vi "ShoulderGetSetpointPreset.vi"(8 "SholdrSetpoints":T1=enum."ShoulderAmp") -> (0 "Setpoint":dbl)   [LabVIEW 2023]
doc: "Gets arm position depending enum value"
uses:
  ShoulderGetSetpointEnum.ctl
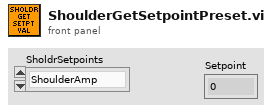
[diagram p1: front panel]
types:
  T1 = typedef "ShoulderGetSetpointEnum.ctl" = enum16{"ShoulderRest", "ShoulderSpeaker", "ShoulderAmp"}
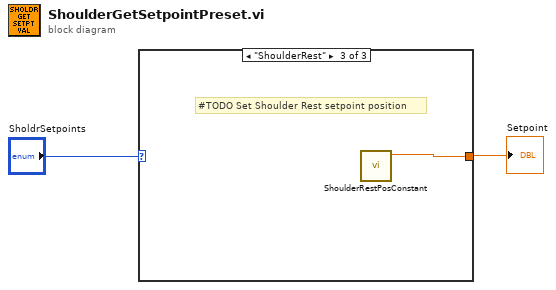
[diagram p0: block diagram]
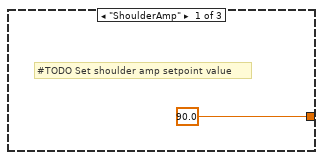
[diagram p2: hidden frame]
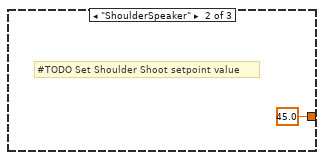
[diagram p3: hidden frame]
diagram:
  n1 = case shown="\"ShoulderRest\"" "SholdrSetpoints" {
    tunnel: [90.0 ("y") 45.0 ("y") w5] -> w1
    frame "ShoulderAmp" {
      # "#TODO Set shoulder amp setpoint value"
    }
    frame "ShoulderSpeaker" {
      # "#TODO Set Shoulder Shoot setpoint value"
    }
    frame "ShoulderRest" {
      # "#TODO Set Shoulder Rest setpoint position"
      n2 = call "ShoulderRestPosConstant.vi"() -> ("RestPosition"=w5:dbl)  [unwired: 11 in]
    }
  }
  "Setpoint" <- w1
